vi "Write Database.vi"(8 "error in (no error)":errorcluster, 10 "Database":refnum<class "Database Interface.lvclass">, 11 "Table Configuration Basic DB in":refnum<class "Table Configuration Basic DB.lvclass">) -> (0 "error out":errorcluster, 3 "Table Configuration Basic DB out":refnum<class "Table Configuration Basic DB.lvclass">)   [LabVIEW 2020, in "Table.lvlib" / "Table Configuration Basic DB.lvclass"]
uses:
  Table Configuration Basic DB.lvclass
  Database Interfaces/Database Interface Class/Database Interface.lvclass
  Table Configuration Basic DB.lvclass/Table Configuration Basic DB.ctl
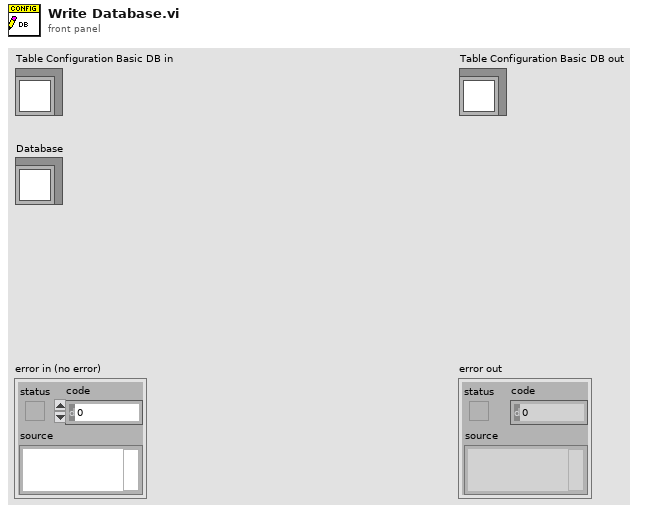
[diagram p1: front panel]
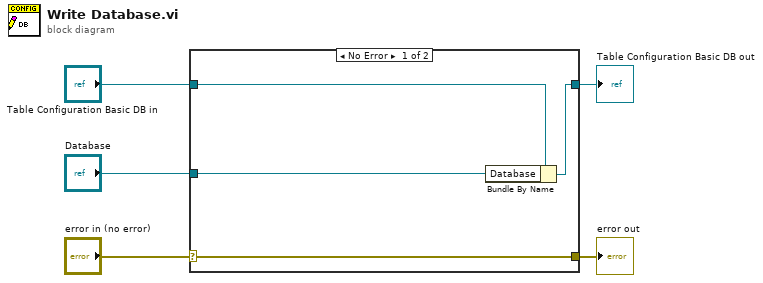
[diagram p0: block diagram]
diagram:
  n1 = case shown="No Error" "error in (no error)" {
    selector: "error in (no error)" -> [w9 w10]
    tunnel: [w9 w10] -> w4
    tunnel: [w7 w11] -> w2
    tunnel: "Table Configuration Basic DB in" -> [w8 w11]
    tunnel: "Database" -> [w6 _]
    frame No Error {
      n2 = Bundle By Name(cluster=w8, "Database"=w6) -> (w7:refnum<class "Table Configuration Basic DB.lvclass">)
    }
    frame Error {
    }
  }
  "error out" <- w4
  "Table Configuration Basic DB out" <- w2
